vi "MKS670_GPIB_set_mode.vi"(6 "wait":dbl format="%#_13g", 7 "mode":enum16{"pressure", "zero", "null", "fulscale"}(ring), 8 "error in":errorcluster, 11 "GPIB in":string) -> (0 "error out":errorcluster, 3 "GPIB out":string, 4 "status":bool)   [LabVIEW 2019]
panel:
  out "string_raw":string
  out "string_fmt":string
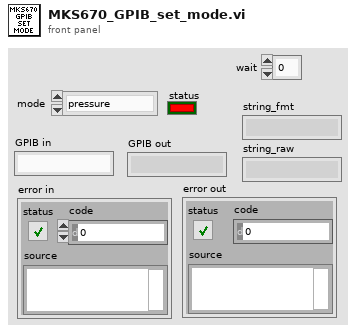
[diagram p1: front panel]
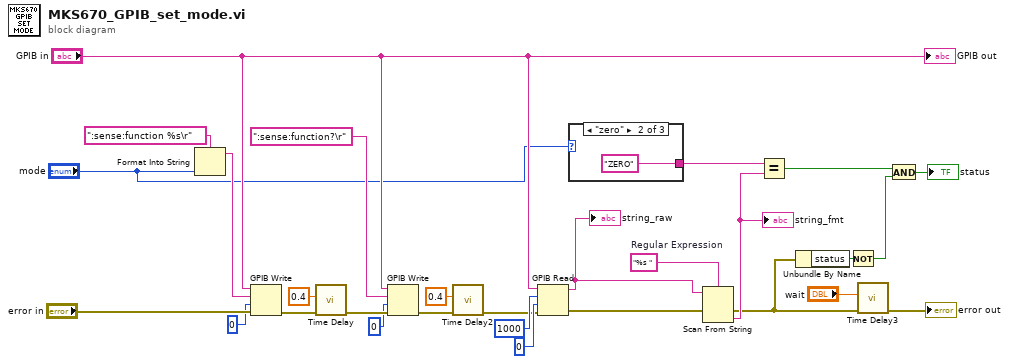
[diagram p0: block diagram]
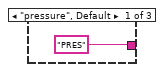
[diagram p2: hidden frame]
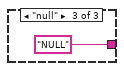
[diagram p3: hidden frame]
diagram:
  w26 = "%s "  # Regular Expression
  n1 = Format Into String(format string=":sense:function %s\r" ("data"), "mode") -> (resulting string=w17:string)  [unwired: 2 in, 1 out]
  n2 = GPIB Write(0:"GPIB in", 1:w17, 2:0, 3:"error in") -> (6:w20:errorcluster)  [unwired: 1 in, 1 out]
  n3 = call "Time Delay"("error in (no error)"=w20, "Delay Time (s)"=0.4) -> ("error out"=w14:errorcluster)  [unwired: 9 in]
  n4 = GPIB Write(0:"GPIB in", 1:":sense:function?\r" ("data"), 2:i16 0 ("mode (0)"), 3:w14) -> (6:w16:errorcluster)  [unwired: 1 in, 1 out]
  n5 = call "Time Delay2"("error in (no error)"=w16, "Delay Time (s)"=0.4) -> ("error out"=w13:errorcluster)  [unwired: 9 in]
  n6 = GPIB Read(0:"GPIB in", 1:1000 ("byte count"), 2:0, 3:w13) -> (5:w25:string, 7:w24:errorcluster)  [unwired: 1 in, 1 out]
  "string_raw" <- w25
  n7 = case shown="\"zero\"" "mode" {
    tunnel: ["PRES" "ZERO" "NULL"] -> w1
    frame "pressure", Default {
    }
    frame "zero" {
    }
    frame "null" {
    }
  }
  n8 = Scan From String(format string=w26, input string=w25, error in=w24) -> (error out=w5:errorcluster, output 1=w9:string)  [unwired: 2 in, 2 out]
  "string_fmt" <- w9
  n9 = Equal?(x=w1, y=w9) -> (x = y?=w8:bool)
  n10 = Unbundle By Name(w5) -> ("status"=w22:bool)
  n11 = Not(x=w22) -> (.not. x?=w7:bool)
  n12 = call "Time Delay3"("error in (no error)"=w5, "Delay Time (s)"="wait") -> ("error out"=→"error out":errorcluster)  [unwired: 9 in]
  n13 = And(x=w8, y=w7) -> (x .and. y?=→"status":bool)
  "GPIB out" <- "GPIB in"
